vi "ULS Sigma Koki.vi"(8 "error in (no error)":errorcluster, 9 "Settings Array":T1(array[cluster]), 10 "Hardware Model":T2={"Controller"=enum."SHOT-304", "X Stage"="", "Y Stage"="", "Z Stage"="", "R Stage"=""}, 11 "IFD in":refnum<class "IFD.lvclass">) -> (0 "error out":errorcluster, 3 "IFD out":refnum<class "IFD.lvclass">)   [LabVIEW 2016, in "IFD.lvclass"]
uses:
  IFD.lvclass
  Tag/IFD_Tag.lvclass/IFD_Tag.ctl
  IFD.lvclass/IFD.ctl
  Tag/IFD_Tag.lvclass
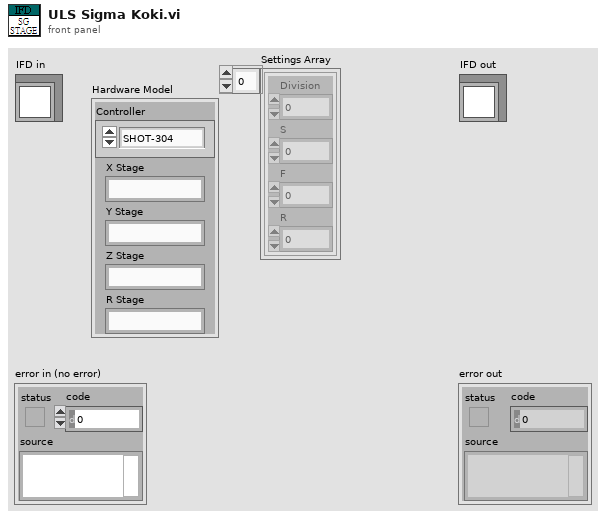
[diagram p1: front panel]
types:
  T1 = cluster{"Division":u8, "S":u32, "F":u32, "R":u32}[]
  T2 = cluster{"Controller":enum32{"GSC-01(PAT)", "SHOT-102", "SHOT-302", "SHOT-602", "SHOT-702", "FINE-503", "SHOT-204", "SHOT-304"}, "X Stage":string, "Y Stage":string, "Z Stage":string, "R Stage":string}
  T3 = enum16{"Undefined(DO NOT USE)", "U8", "ASCII", "U16", "U32", "RATIONAL", "I8", "Undefined 8 bit", "I16", "I32", "SRATIONAL", "SGL", "DBL"}
  T4 = enum32{"GSC-01(PAT)", "SHOT-102", "SHOT-302", "SHOT-602", "SHOT-702", "FINE-503", "SHOT-204", "SHOT-304"}
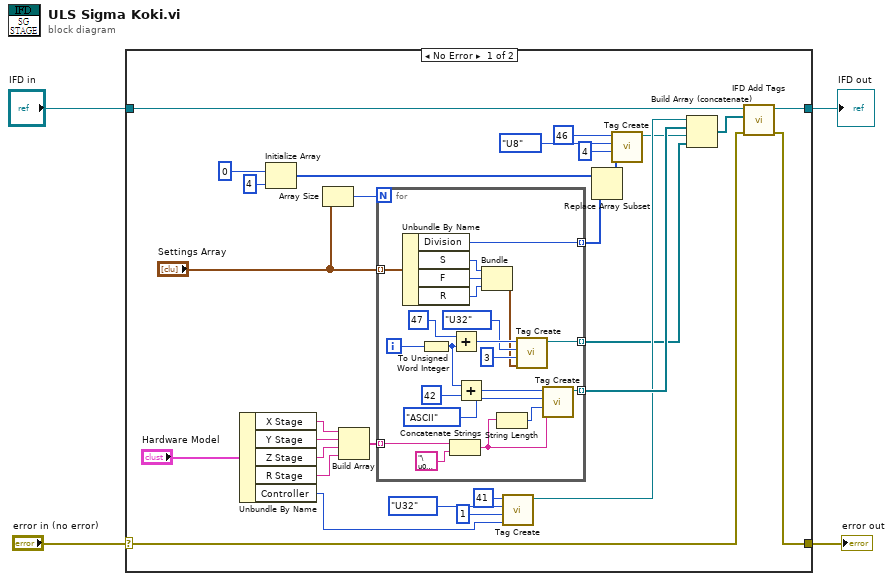
[diagram p0: block diagram]
diagram:
  n1 = case shown="No Error" "error in (no error)" {
    selector: "error in (no error)" -> [w30 w56]
    tunnel: [w33 w56] -> w3
    tunnel: [w32 w55] -> w1
    tunnel: "IFD in" -> [w31 w55]
    frame No Error {
      n2 = Unbundle By Name("Hardware Model") -> ("X Stage"=w27:string, "Y Stage"=w26:string, "Z Stage"=w25:string, "R Stage"=w24:string, "Controller"=w8:T4)
      n3 = Initialize Array(u8 0, 4 ("dimension size")) -> (w7:u8[])
      n4 = Array Size(array="Settings Array") -> (size(s)=w23:i32)
      n5 = Build Array(w27, w26, w25, w24) -> (w21:string[])
      n6 = for {
        N: w23 -> [_]
        tunnel: "Settings Array" -> [w54] mode=indexing
        tunnel: w21 -> [w40] mode=indexing
        tunnel: [w45] -> w18 mode=indexing
        tunnel: [w36] -> w20 mode=indexing
        tunnel: [w34] -> w6 mode=indexing
        i -> [w35]
        n7 = Unbundle By Name(w54) -> ("Division"=w34:u8, "S"=w50:u32, "F"=w51:u32, "R"=w49:u32)
        n8 = To Unsigned Word Integer(number=w35) -> (unsigned 16bit integer=w43:u16)
        n9 = Concatenate Strings(w40, "\u0000") -> (w37:string)
        n10 = Add(x=u16 47 ("Tag ID"), y=w43) -> (x+y=w52:u16)
        n11 = Add(x=w43, y=u16 42 ("Tag ID")) -> (x+y=w42:u16)
        n12 = Bundle("S"=w50, "F"=w51, "R"=w49) -> (w46:cluster{"S":u32, "F":u32, "R":u32})  [unwired: 1 in]
        n13 = String Length(string=w37) -> (length=w38:i32)
        n14 = call "Tag Create.vi"("Data"=w46, "Data Count"=u32 3, "Data Type"=T3."U32", "Tag ID"=w52) -> ("IFD_Tag out"=w45:refnum<class "IFD_Tag.lvclass">)  [unwired: 7 in]
        n15 = call "Tag Create.vi"("Data"=w37, "Data Count"=w38, "Data Type"=T3."ASCII", "Tag ID"=w42) -> ("IFD_Tag out"=w36:refnum<class "IFD_Tag.lvclass">)  [unwired: 7 in]
      }
      n16 = call "Tag Create.vi"("Data"=w8, "Data Count"=u32 1, "Data Type"=T3."U32", "Tag ID"=u16 41) -> ("IFD_Tag out"=w19:refnum<class "IFD_Tag.lvclass">)  [unwired: 7 in]
      n17 = Replace Array Subset(array=w7, new element=w6) -> (w5:u8[])  [unwired: 1 in]
      n18 = call "Tag Create.vi"("Data"=w5, "Data Count"=u32 4, "Data Type"=T3."U8", "Tag ID"=u16 46) -> ("IFD_Tag out"=w12:refnum<class "IFD_Tag.lvclass">)  [unwired: 7 in]
      n19 = Build Array (concatenate)(w19, w20, w12, w18) -> (w28:refnum<class "IFD_Tag.lvclass">[])
      n20 = call "IFD Add Tags.vi"("error in (no error)"=w30, "Tag(s)"=w28, "IFD in"=w31) -> ("error out"=w33:errorcluster, "IFD out"=w32:refnum<class "IFD.lvclass">)  [unwired: 7 in]
    }
    frame Error {
    }
  }
  "error out" <- w3
  "IFD out" <- w1
